vi "FPGA_DIOWritePWMPeriodScale.vi"(8 "error in (no error)":errorcluster, 9 "PWMPeriodScale":u8, 10 "PWMChannel":T1, 11 "DIODeviceRef In":T2) -> (0 "error out":errorcluster, 3 "DIODeviceRef Out":T2)   [LabVIEW 2017]
uses:
  <vilib>/Rock Robotics/SystemInterfaces/DIO/FPGA_DIODevRef.ctl
  <vilib>/Rock Robotics/SystemInterfaces/DIO/FPGA_DIOPWMChannel.ctl
  <vilib>/Rock Robotics/SystemInterfaces/System/FPGA_SystemFPGA Ref Global.vi
  <vilib>/Utility/error.llb/Error Cluster From Error Code.vi
  <vilib>/rvi/errors/niLvFpgaAdjustHostInterfaceError.vi
  <vilib>/rvi/interface/nirviReadWriteControl/nirviReadWriteControl.xnode
  <vilib>/Rock Robotics/SystemInterfaces/System/FPGA_SystemFRC FPGA Ref.ctl
  <vilib>/rvi/interface/Simulation/niFpgaSimulationCallBeginRW.vi
  NiFpgaLv.dll
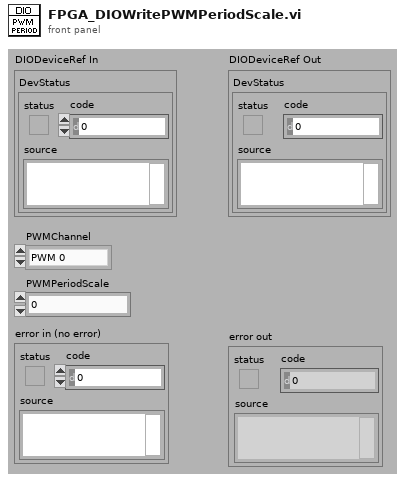
[diagram p1: front panel]
types:
  T1 = typedef "FPGA_DIOPWMChannel.ctl" = enum8{"PWM 0", "PWM 1", "PWM 2", "PWM 3", "PWM 4", "PWM 5", "PWM 6", "PWM 7", "PWM 8", "PWM 9", "PWM MXP 0", "PWM MXP 1", "PWM MXP 2", "PWM MXP 3", "PWM MXP 4", "PWM MXP 5", "PWM MXP 6", "PWM MXP 7", "PWM MXP 8", "PWM MXP 9", "Invalid"}
  T2 = typedef "FPGA_DIODevRef.ctl" = cluster{"DevStatus":errorcluster}
  T3 = typedef "FPGA_SystemFRC FPGA Ref.ctl" = refnum<k20>
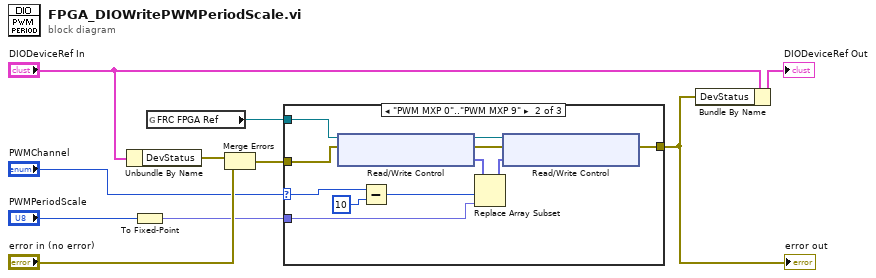
[diagram p0: block diagram]
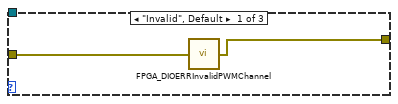
[diagram p2: hidden frame]
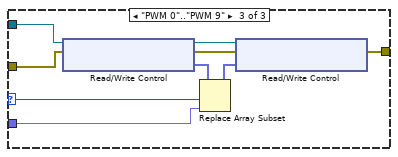
[diagram p3: hidden frame]
diagram:
  n1 = Unbundle By Name("DIODeviceRef In") -> ("DevStatus"=w3:errorcluster)
  n2 = To Fixed-Point(number="PWMPeriodScale") -> (fixed-point=w5:fxp<+,2,2>)  [unwired: 1 in]
  n3 = global read "FPGA_SystemFPGA Ref Global.vi" "FRC FPGA Ref"() -> (w4:T3)
  n4 = Merge Errors(w3, "error in (no error)") -> (w2:errorcluster)
  n5 = case shown="\"PWM MXP 0\"..\"PWM MXP 9\"" "PWMChannel" {
    selector: "PWMChannel" -> [_ w18 w27]
    tunnel: w2 -> [w12 w16 w25]
    tunnel: [w11 w22 w31] -> w7
    tunnel: w5 -> [_ w19 w28]
    tunnel: w4 -> [_ w15 w24]
    frame "Invalid", Default {
      n6 = call <vilib>:"FPGA_DIOERRInvalidPWMChannel.vi"("error in (no error)"=w12) -> ("error out"=w11:errorcluster)
    }
    frame "PWM MXP 0".."PWM MXP 9" {
      n7 = xnode "Read/Write Control"("FPGA VI Reference In"=w15, "error in"=w16) -> ("FPGA VI Reference Out"=w23:T3, "error out"=w17:errorcluster, "PWM.PeriodScaleMXP"=w21:fxp<+,2,2>[])
      n8 = Subtract(x=w18, y=u8 10 ("Numeric")) -> (x-y=w14:u8)
      n9 = Replace Array Subset(array=w21, new element=w19, index=w14) -> (w20:fxp<+,2,2>[])
      n10 = xnode "Read/Write Control"("FPGA VI Reference In"=w23, "error in"=w17, "PWM.PeriodScaleMXP"=w20) -> ("error out"=w22:errorcluster)  [unwired: 1 out]
    }
    frame "PWM 0".."PWM 9" {
      n11 = xnode "Read/Write Control"("FPGA VI Reference In"=w24, "error in"=w25) -> ("FPGA VI Reference Out"=w32:T3, "error out"=w26:errorcluster, "PWM.PeriodScaleHdr"=w30:fxp<+,2,2>[])
      n12 = Replace Array Subset(array=w30, new element=w28, index=w27) -> (w29:fxp<+,2,2>[])
      n13 = xnode "Read/Write Control"("FPGA VI Reference In"=w32, "error in"=w26, "PWM.PeriodScaleHdr"=w29) -> ("error out"=w31:errorcluster)  [unwired: 1 out]
    }
  }
  "error out" <- w7
  n14 = Bundle By Name(cluster="DIODeviceRef In", "DevStatus"=w7) -> (→"DIODeviceRef Out":T2)
